vi "cg_Brent Search Powell Prep.vi"(4 "ZEPS":dbl format="%.2f", 6 "e":dbl format="%.2f", 7 "c (start)":dbl format="%.2f", 8 "tol":dbl format="%.2f", 9 "a (start)":dbl format="%.2f", 10 "b (start)":dbl format="%.2f") -> (0 "value a":dbl format="%.2f", 1 "value b":dbl format="%.2f", 2 "convergence?":bool, 3 "tol2":dbl format="%.2f", 5 "value c":dbl format="%.2f")   [LabVIEW 2018, in "NI_Gmath.lvlib"]
uses:
  NI_Gmath.lvlib
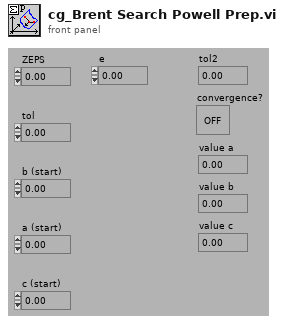
[diagram p1: front panel]
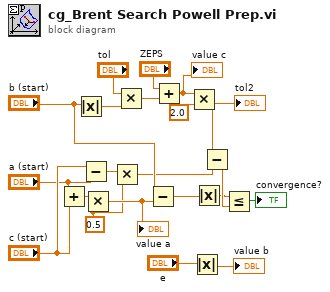
[diagram p0: block diagram]
diagram:
  w3 = 0.5
  n1 = Add(x="a (start)", y="c (start)") -> (x+y=w1:dbl)
  n2 = Absolute Value(x="b (start)") -> (abs(x)=w4:dbl)
  n3 = Subtract(x="c (start)", y="a (start)") -> (x-y=w2:dbl)
  n4 = Multiply(x=w1, y=w3) -> (x*y=w18:dbl)
  "value a" <- w18
  n5 = Multiply(x=w2, y=w3) -> (x*y=w10:dbl)
  n6 = Multiply(x="tol", y=w4) -> (x*y=w6:dbl)
  n7 = Subtract(x="b (start)", y=w18) -> (x-y=w11:dbl)
  n8 = Add(x="ZEPS", y=w6) -> (x+y=w17:dbl)
  "value c" <- w17
  n9 = Multiply(x=w17, y=2.0) -> (x*y=w9:dbl)
  "tol2" <- w9
  n10 = Absolute Value(x="e") -> (abs(x)=→"value b":dbl)
  n11 = Absolute Value(x=w11) -> (abs(x)=w12:dbl)
  n12 = Subtract(x=w9, y=w10) -> (x-y=w13:dbl)
  n13 = Less Or Equal?(x=w12, y=w13) -> (x <= y?=→"convergence?":bool)
